vi "ziExample-CNT.vi"() -> ()   [LabVIEW 2009]
doc: "Control a Zurich instrument device via the LabOne Labview API. \nRequirements: Zurich Instruments MFLI, HF2 or UHFLI \nThe example streams the counter data of a trigger input.\n\n© Zurich Instruments AG, www.zhinst.com"
uses:
  <instrlib>/Zurich Instruments LabOne/Public/Configure/ziSetValueDoubleArray.vi
  <instrlib>/Zurich Instruments LabOne/Public/Utility/ziTicksToS_vector.vi
  <instrlib>/Zurich Instruments LabOne/Public/Data/ziGetEventCntSample.vi
  <instrlib>/Zurich Instruments LabOne/Zurich Instruments LabOne.lvlib
panel:
  out "data":cluster{"Timestamp(s)":dbl[], u32[]}
  out "All Values (V)":cluster{"Timestamp(s)":dbl[], i32[]}(graph)
  out "Error Out":errorcluster
  in  "Address":string="DEV"
  out "Selected Device":string
  out "Unexpected Node":string[](array[string])
  in  "stop":bool=TRUE
  # "ziExample-CNT.vi\nRequirements:  UHFLI + CNT Option\nsee block diagram for VI description"
  # "Tested Instruments:\n- UHF"
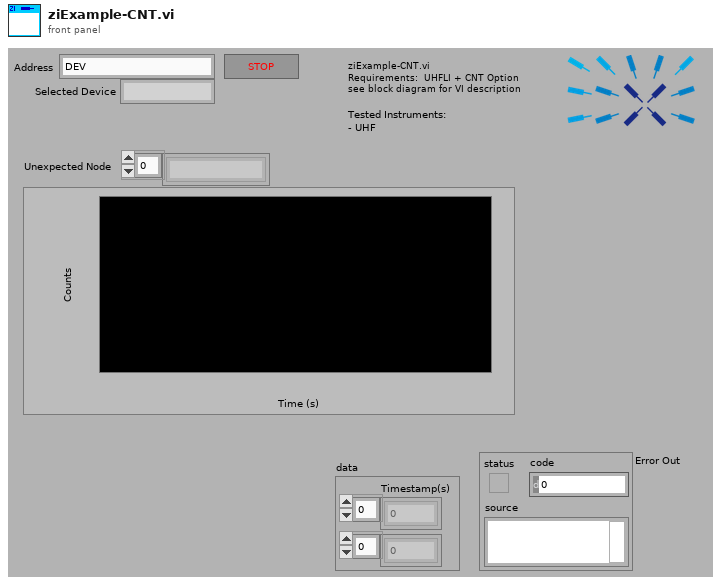
[diagram p1: front panel]
types:
  T1 = typedef "Zurich Instruments LabOne.lvlib/ziTypeHandle.ctl" = cluster{"handleValid":bool, "Conn":u64, "Path Prefix":string, "Handle":u64, "Connected":bool, "Clockbase(s)":dbl}
  T2 = typedef "Zurich Instruments LabOne.lvlib/ziTypeCounterSample.ctl" = cluster{"Timestamps (ticks)":u64[], "Counter":i32[], "ID":u16[]}
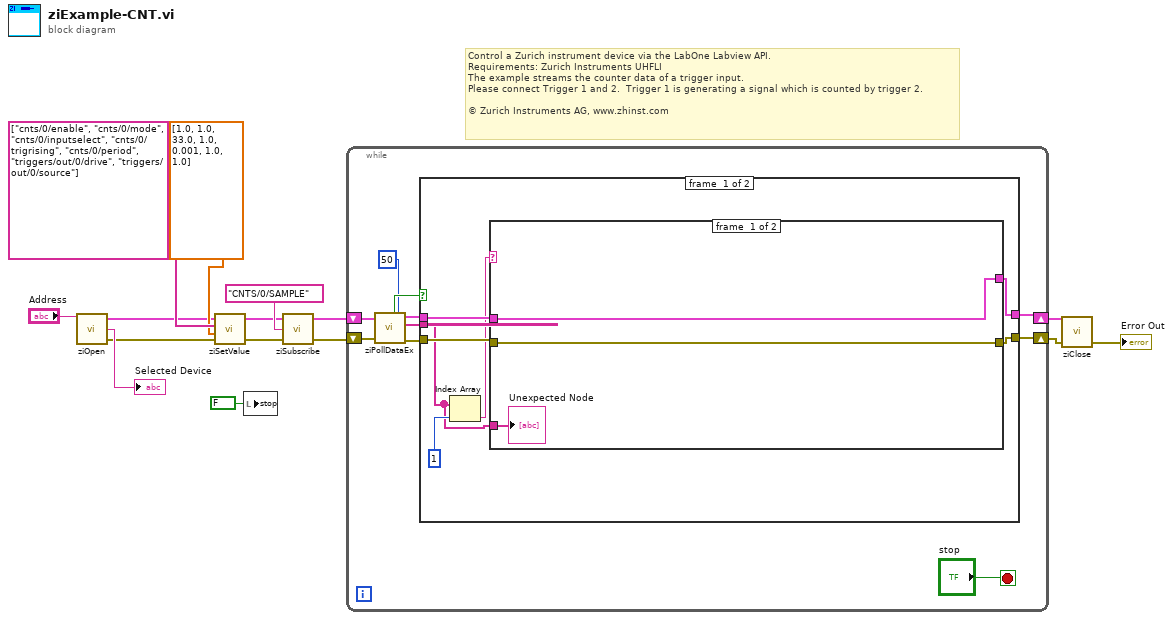
[diagram p0: block diagram]
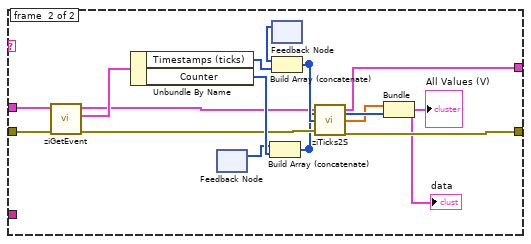
[diagram p2: hidden frame]
diagram:
  # "Control a Zurich instrument device via the LabOne Labview API. \nRequirements: Zurich Instruments UHFLI  \nThe example streams the counter data of a trigger input.\nPlease connect Trigger 1 and 2.  Trigger 1 is generating a signal which is counted by trigger 2.\n\n© Zurich Instruments AG, www.zhinst.com"
  n1 = call <instrlib>:"ziOpen.vi"("Address"="Address") -> ("Error Out"=w2:errorcluster, "Selected Device"=→"Selected Device":string, "HandleOut"=w1:T1)  [unwired: 3 in]
  n2 = call-poly <instrlib>:"ziSetValue.vi"("Error In"=w2, "Values"=dbl[] [1.0, 1.0, 33.0, 1.0, 0.001, 1.0, 1.0], "Paths"=string[] ["cnts/0/enable", "cnts/0/mode", "cnts/0/inputselect", "cnts/0/trigrising", "cnts/0/period", "triggers/out/0/drive", "triggers/out/0/source"], "Handle In"=w1) -> ("Error Out"=w4:errorcluster, "Handle Out"=w3:T1)  [unwired: 1 in]
  n3 = local write "stop"(FALSE ("stop")) -> ()
  n4 = call <instrlib>:"ziSubscribe.vi"("error in"=w4, "Path ()"="CNTS/0/SAMPLE", "Handle In"=w3) -> ("error out"=w7:errorcluster, "Handle Out"=w13:T1)  [unwired: 1 in]
  n5 = while {
    shift-right: [w17] -> w14
    shift-left: w13 -> [w24]
    shift-right: [w16] -> w15
    shift-left: w7 -> [w25]
    stop <- "stop" stop-if-true
    n6 = call <instrlib>:"ziPollDataEx.vi"("error in"=w25, "Timeout ms (50)"=50 ("TimeOut ms (50)"), "Handle In"=w24) -> ("error out"=w18:errorcluster, "PathArray"=w22:string[], "Handle Out"=w19:T1, "Timed Out"=w23:bool)  [unwired: 1 in, 4 out]
    n7 = case shown="False" w23 {
      tunnel: w22 -> [w26 _]
      tunnel: w19 -> [w32 w52]
      tunnel: w18 -> [w31 w51]
      tunnel: [w30 w52] -> w17
      tunnel: [w29 w51] -> w16
      frame #0 {
        n8 = Index Array(array=w26, index=1) -> (element=w27:string)
        n9 = case shown="\"CNTS\"" w27 {
          tunnel: w32 -> [w35 w50]
          tunnel: w31 -> [w34 w49]
          tunnel: [w35 w41] -> w30
          tunnel: [w34 w39] -> w29
          tunnel: w26 -> [w33 _]
          frame #0 {
            "Unexpected Node" <- w33
          }
          frame #1 {
            n10 = call-poly <instrlib>:"ziGetEvent.vi"("Error In"=w49, "Handle In"=w50) -> ("Error Out"=w40:errorcluster, "Cnt Sample Out"=w48:T2, "Handle Out"=w42:T1)  [unwired: 7 in]
            n11 = Unbundle By Name(w48) -> ("Timestamps (ticks)"=w47:u64[], "Counter"=w45:i32[])
            n12 = feedback #1() -> (w44:i32[])  [unwired: 1 in]
            n13 = Build Array (concatenate)(w44, w45) -> (w38:i32[])
            n14 = feedback #2() -> (w46:u64[])  [unwired: 1 in]
            n15 = Build Array (concatenate)(w46, w47) -> (w43:u64[])
            n16 = call-poly <instrlib>:"ziTicks2S.vi"("Error In"=w40, "Timestamp (ticks)"=w43, "Handle In"=w42) -> ("Error Out"=w39:errorcluster, "Timestamp(s)"=w37:dbl[], "Handle Out"=w41:T1)
            n17 = Bundle("Timestamp(s)"=w37, w38) -> (→"All Values (V)" →"data":cluster{"Timestamp(s)":dbl[], i32[]})  [unwired: 1 in]
          }
        }
      }
      frame #1 {
      }
    }
  }
  n18 = call <instrlib>:"ziClose.vi"("Error In"=w15, "Handle In"=w14) -> ("Error Out"=→"Error Out":errorcluster)  [unwired: 2 in, 1 out]
